vi "Item_Init.vi"(11 "Object":T1) -> ()   [LabVIEW 2020, in "LUnit Project Provider.lvlib"]
uses:
  <resource>/Framework/Providers/API/ItemRef.ctl
  LUnit Project Provider.lvlib
  Framework/Icon Decorator/Icon Decorator.lvclass
panel:
  out "error out":errorcluster
  in  "error in":errorcluster
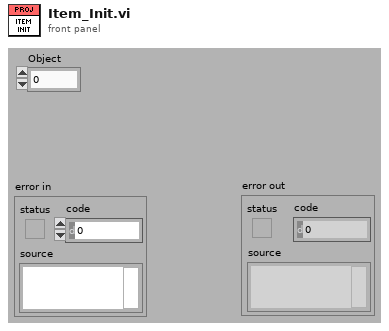
[diagram p1: front panel]
types:
  T1 = typedef "ItemRef.ctl" = u64
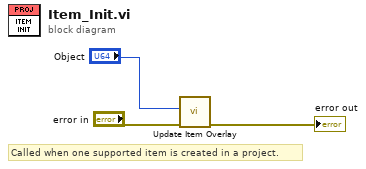
[diagram p0: block diagram]
diagram:
  # "Called when one supported item is created in a project."
  n1 = call "Update Item Overlay.vi"("error in (no error)"="error in", "Item"="Object") -> ("error out"=→"error out":errorcluster)  [unwired: 8 in, 1 out]
